vi "Replace Values Array One Timestamp.vi"(4 "Values (new)":u8[](array[numeric]), 6 "Timestamps (new)":u64, 7 "#bytes per timestamp":i32, 9 "index":i32, 10 "Values (buffered)":u8[](array[numeric]), 11 "Timestamps (buffered)":u64[](array[numeric])) -> (2 "Values (buffered)":u8[](array[numeric]), 3 "Timestamps (buffered)":u64[](array[numeric]))   [LabVIEW 2021, in "Ring Buffer Time Series Data.lvlib"]
uses:
  Ring Buffer Time Series Data.lvlib
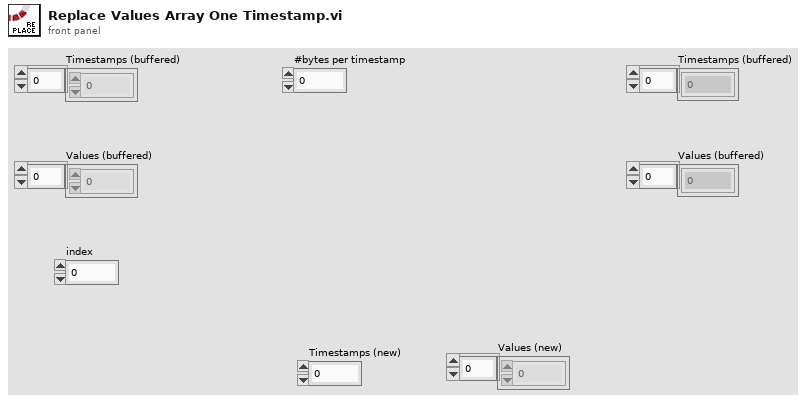
[diagram p1: front panel]
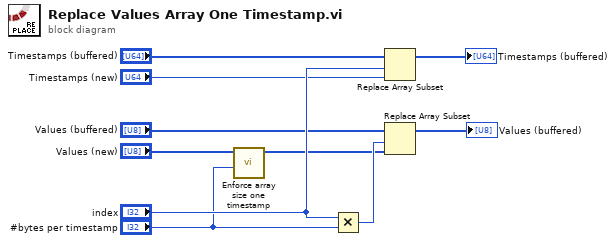
[diagram p0: block diagram]
diagram:
  n1 = call "Enforce array size one timestamp.vi"("#bytes per timestamp"="#bytes per timestamp", "Values (new)"="Values (new)") -> ("Values (new) [padded]"=w2:u8[])  [unwired: 9 in]
  n2 = Multiply(x="index", y="#bytes per timestamp") -> (x*y=w6:i32)
  n3 = Replace Array Subset(array="Timestamps (buffered)", new element="Timestamps (new)", index="index") -> (→"Timestamps (buffered)":u64[])
  n4 = Replace Array Subset(array="Values (buffered)", new element=w2, index=w6) -> (→"Values (buffered)":u8[])
